vi "Add Client Protocol Header.vi"(8 "error in (no error)":errorcluster, 11 "WebSocket Client in":refnum<class "WebSocket Client.lvclass">) -> (0 "error out":errorcluster, 3 "WebSocket Client out":refnum<class "WebSocket Client.lvclass">)   [LabVIEW 2021, in "WebSockets.lvlib" / "WebSocket Client.lvclass"]
doc: "If supported protocols have been specified, adds the Sec-WebSocket-Protocol header to the send headers.\nWebSockets 2.0.1.40\nSam Sharp - MediaMongrels Ltd\nCopyright (c) 2019, MediaMongrels Ltd"
uses:
  WebSocket Client.lvclass
  D:/my_projects/projects/Algorithms/Labview/21/WebSockets/WebSockets/WebSocket/WebSocket.lvclass
  WebSocket/WebSocket.lvclass/WebSocket.ctl
  WebSocket/Read Protocols.vi
  WebSocket/WebSocket.lvclass
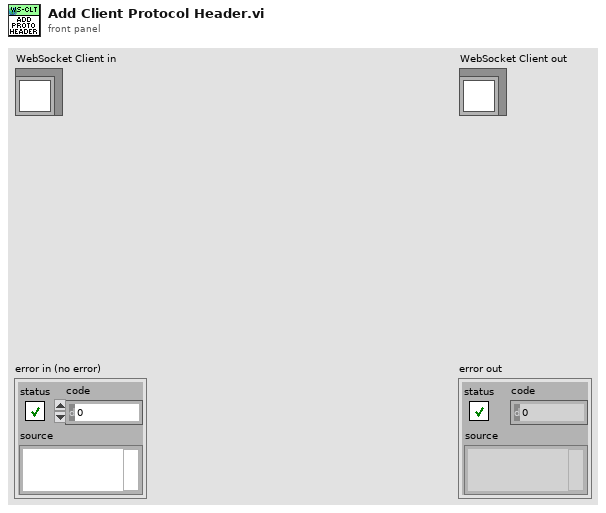
[diagram p1: front panel]
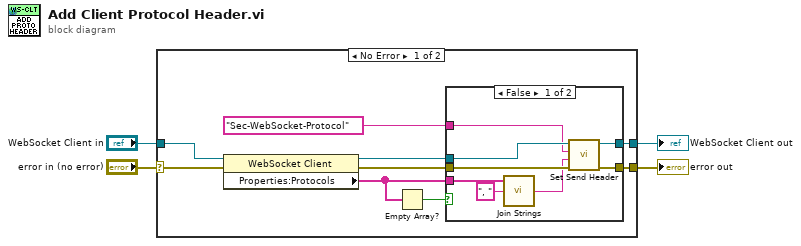
[diagram p0: block diagram]
diagram:
  n1 = case shown="No Error" "error in (no error)" {
    selector: "error in (no error)" -> [w12 w25]
    tunnel: [w8 w25] -> w3
    tunnel: [w9 w24] -> w1
    tunnel: "WebSocket Client in" -> [w13 w24]
    frame No Error {
      n2 = property class="WebSocket Client"(reference=w13, error in=w12) -> (reference out=w10:refnum<class "WebSocket Client.lvclass">, error out=w11:errorcluster, "Properties:Protocols"=w7:string[])
      n3 = Empty Array?(array=w7) -> (empty?=w6:bool)
      n4 = case shown="False" w6 {
        tunnel: w11 -> [w21 w22]
        tunnel: w10 -> [w20 w23]
        tunnel: [w19 w23] -> w9
        tunnel: [w18 w22] -> w8
        tunnel: w7 -> [w16 _]
        tunnel: "Sec-WebSocket-Protocol" ("Name") -> [w15 _]
        frame False {
          n5 = call <vilib>:"Join Strings.vi"("Separator (,)"=", ", "Strings In"=w16) -> ("String"=w17:string)  [unwired: 1 in]
          n6 = call "Set Send Header.vi"("error in (no error)"=w21, "Value"=w17, "Name"=w15, "WebSockets in"=w20) -> ("error out"=w18:errorcluster, "WebSockets out"=w19:refnum<class "WebSocket Client.lvclass">)  [unwired: 6 in]
        }
        frame True {
        }
      }
    }
    frame Error {
    }
  }
  "error out" <- w3
  "WebSocket Client out" <- w1
